vi "test_VerifyVIsNotBroken.vi"() -> ()   [LabVIEW 2020]
panel:
  out "result":string
  out "pass":bool
  out "error out":errorcluster
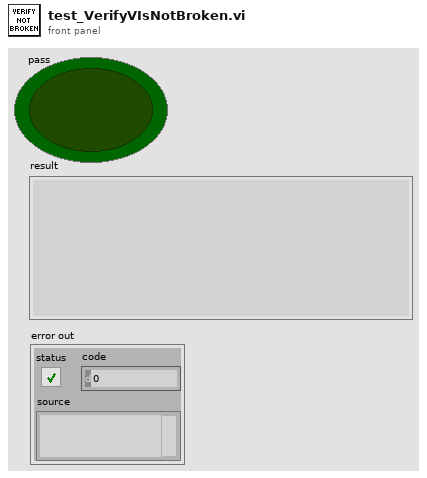
[diagram p1: front panel]
types:
  T1 = enum32{"Bad", "Idle", "Run top level", "Running"}
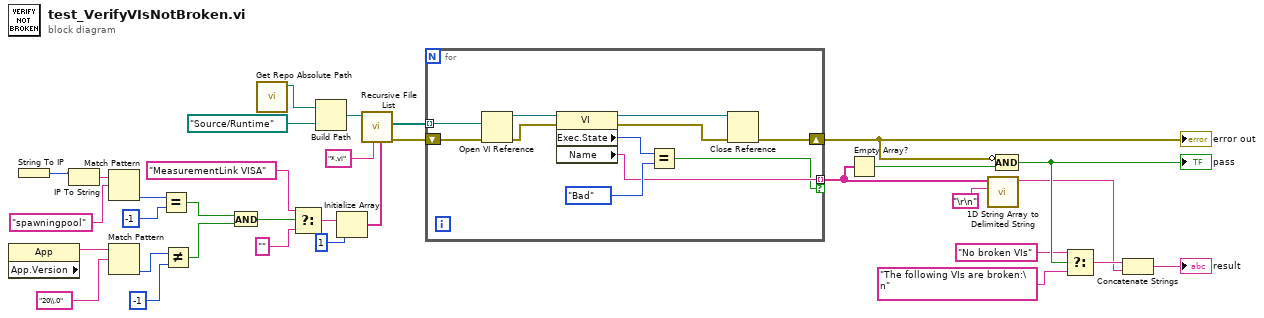
[diagram p0: block diagram]
diagram:
  n1 = property class="App"() -> ("App.Version"=w17:string)  [unwired: 2 in, 2 out]
  n2 = String To IP() -> (0:w13:u32)  [unwired: 1 in]
  n3 = IP To String(2:w13) -> (0:w12:string)  [unwired: 1 in]
  n4 = Match Pattern(string=w12, regular expression="spawningpool" ("y")) -> (offset past match=w10:i32)  [unwired: 1 in, 3 out]
  n5 = Match Pattern(string=w17, regular expression="20\\.0") -> (offset past match=w15:i32)  [unwired: 1 in, 3 out]
  n6 = Equal?(x=w10, y=-1) -> (x = y?=w2:bool)
  n7 = Not Equal?(x=w15, y=-1) -> (x != y?=w1:bool)
  n8 = And(x=w2, y=w1) -> (x .and. y?=w8:bool)
  n9 = call "Get Repo Absolute Path.vi"() -> ("repo path"=w21:path)  [unwired: 11 in]
  n10 = Select(t="MeasurementLink VISA", s=w8, f="") -> (s? t:f=w7:string)
  n11 = Build Path(base path=w21, name or relative path=path "Source/Runtime") -> (appended path=w20:path)
  n12 = Initialize Array(w7, 1 ("dimension size")) -> (w5:string[])
  n13 = call <vilib>:"Recursive File List.vi"("Folders to Exclude"=w5, "pattern"="*.vi", "Folder Path"=w20) -> ("error out"=w23:errorcluster, "All Files in Dir"=w18:path[])  [unwired: 4 in, 3 out]
  n14 = for {
    tunnel: w18 -> [w38] mode=indexing
    shift-right: [w44] -> w30
    shift-left: w23 -> [w39]
    tunnel: [w35] -> w32 mode=indexing if=w34
    n15 = Open VI Reference(vi path=w38, error in (no error)=w39) -> (vi reference=w42:refnum<vi>, error out=w43:errorcluster)  [unwired: 4 in]
    n16 = property class="VI"(reference=w42, error in=w43) -> (reference out=w41:refnum<vi>, error out=w40:errorcluster, "Exec.State"=w37:T1, "Name"=w35:string)
    n17 = Equal?(x=w37, y=T1."Bad") -> (x = y?=w34:bool)
    n18 = Close Reference(reference=w41, error in (no error)=w40) -> (error out=w44:errorcluster)
  }
  "error out" <- w30
  n19 = Empty Array?(array=w32) -> (empty?=w31:bool)
  n20 = call <vilib>:"1D String Array to Delimited String.vi"("delimiter"="\r\n", "string array"=w32) -> ("delimited string"=w25:string)  [unwired: 9 in]
  n21 = Compound Arithmetic op=AND(invert w30, w31) -> (w29:bool)
  "pass" <- w29
  n22 = Select(t="No broken VIs", s=w29, f="The following VIs are broken:\n") -> (s? t:f=w26:string)
  n23 = Concatenate Strings(w26, w25) -> (→"result":string)
